vi "HintfullPicture.vi"(8 "length(y)":i32, 9 "width(x)":i32, 10 "image data":T1) -> (2 "new picture":picture)   [LabVIEW 2014]
uses:
  <vilib>/picture/picture.llb/imagedata.ctl
panel:
  in  "stop":bool
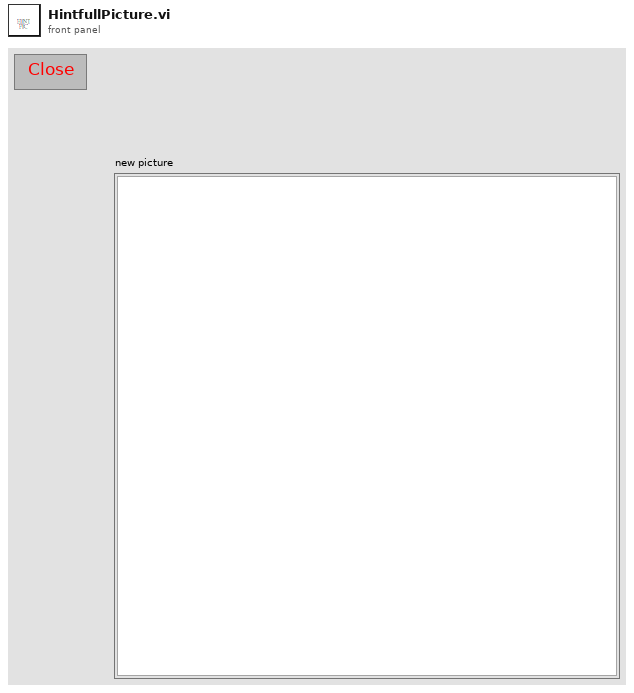
[diagram p1: front panel]
types:
  T1 = typedef "imagedata.ctl" = cluster{"image type":i32, "image depth":i32, "image":u8[], "mask":u8[], "colors":u32[], "Rectangle":cluster{"left":i16, "top":i16, "right":i16, "bottom":i16}}
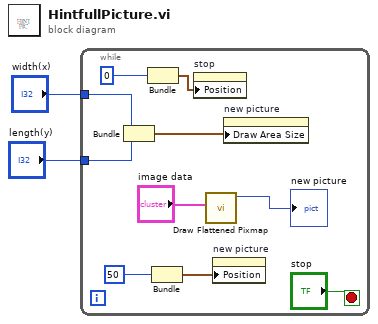
[diagram p0: block diagram]
diagram:
  n1 = while {
    tunnel: "length(y)" -> [w8]
    tunnel: "width(x)" -> [w7]
    stop <- "stop" stop-if-true
    w4 = 0
    w10 = 50
    n2 = Bundle("width(x)"=w7, "length(y)"=w8) -> (w9:cluster{"width(x)":i32, "length(y)":i32})  [unwired: 1 in]
    n3 = Bundle(w4, w4) -> (w3:cluster{i32, i32})  [unwired: 1 in]
    n4 = Bundle(w10, w10) -> (w11:cluster{i32, i32})  [unwired: 1 in]
    n5 = property on="stop" class="Bool"("Position"=w3) -> ()  [unwired: 2 in, 2 out]
    n6 = call <vilib>:"Draw Flattened Pixmap.vi"("image data"="image data") -> ("new picture"=→"new picture":picture)  [unwired: 8 in]
    n7 = property on="new picture" class="Pict"("Position"=w11) -> ()  [unwired: 2 in, 2 out]
    n8 = property on="new picture" class="Pict"("Draw Area Size"=w9) -> ()  [unwired: 2 in, 2 out]
  }
